vi "Solver.vi"(10 "Word List":string[](array[string]), 11 "Word Search Grid":string[][](array[string])) -> (3 "Solutions":T1)   [LabVIEW 2023]
uses:
  support/Solutions--map.ctl
  support/Letter Index--cluster.ctl
panel:
  # "Implement your Word Search challenge solution in this VI. Do not change the connector pane of this VI."
  # "Letters will always be ALL CAPS."
  # "Words will always be ALL CAPS."
  # "The Word Search Grid contains the 2D array of letters in which all words in the Word List appear. Words can appear forwards, backwards, up, down, and diagonally in any direction.\n\nThe Solutions map will contain one entry per item in the Word List. The map elements are:\n\nWord: The word from the Word List.\nLetter Indices: The row/column indices into the Word Search Grid for each letter (in order) in the word."
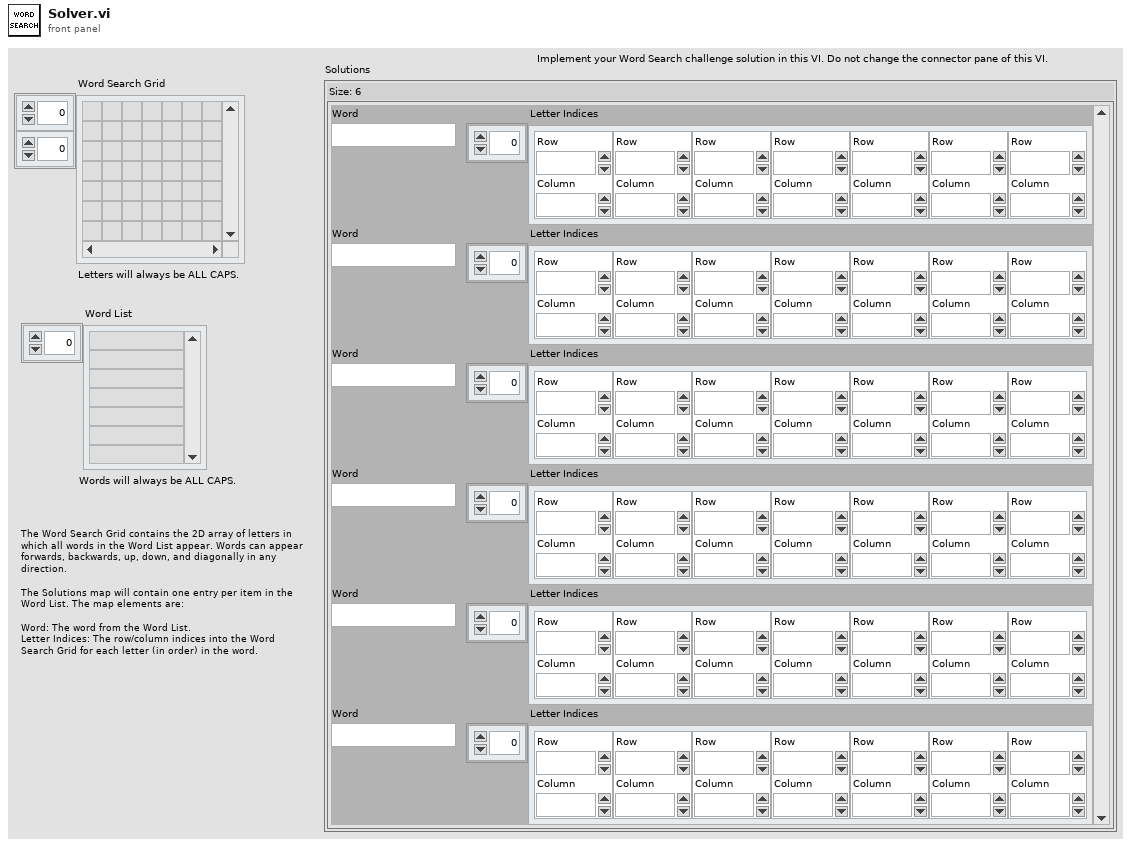
[diagram p1: front panel]
types:
  T1 = typedef "Solutions--map.ctl" = map{string, T2[]}
  T2 = typedef "Letter Index--cluster.ctl" = cluster{"Row":i32, "Column":i32}
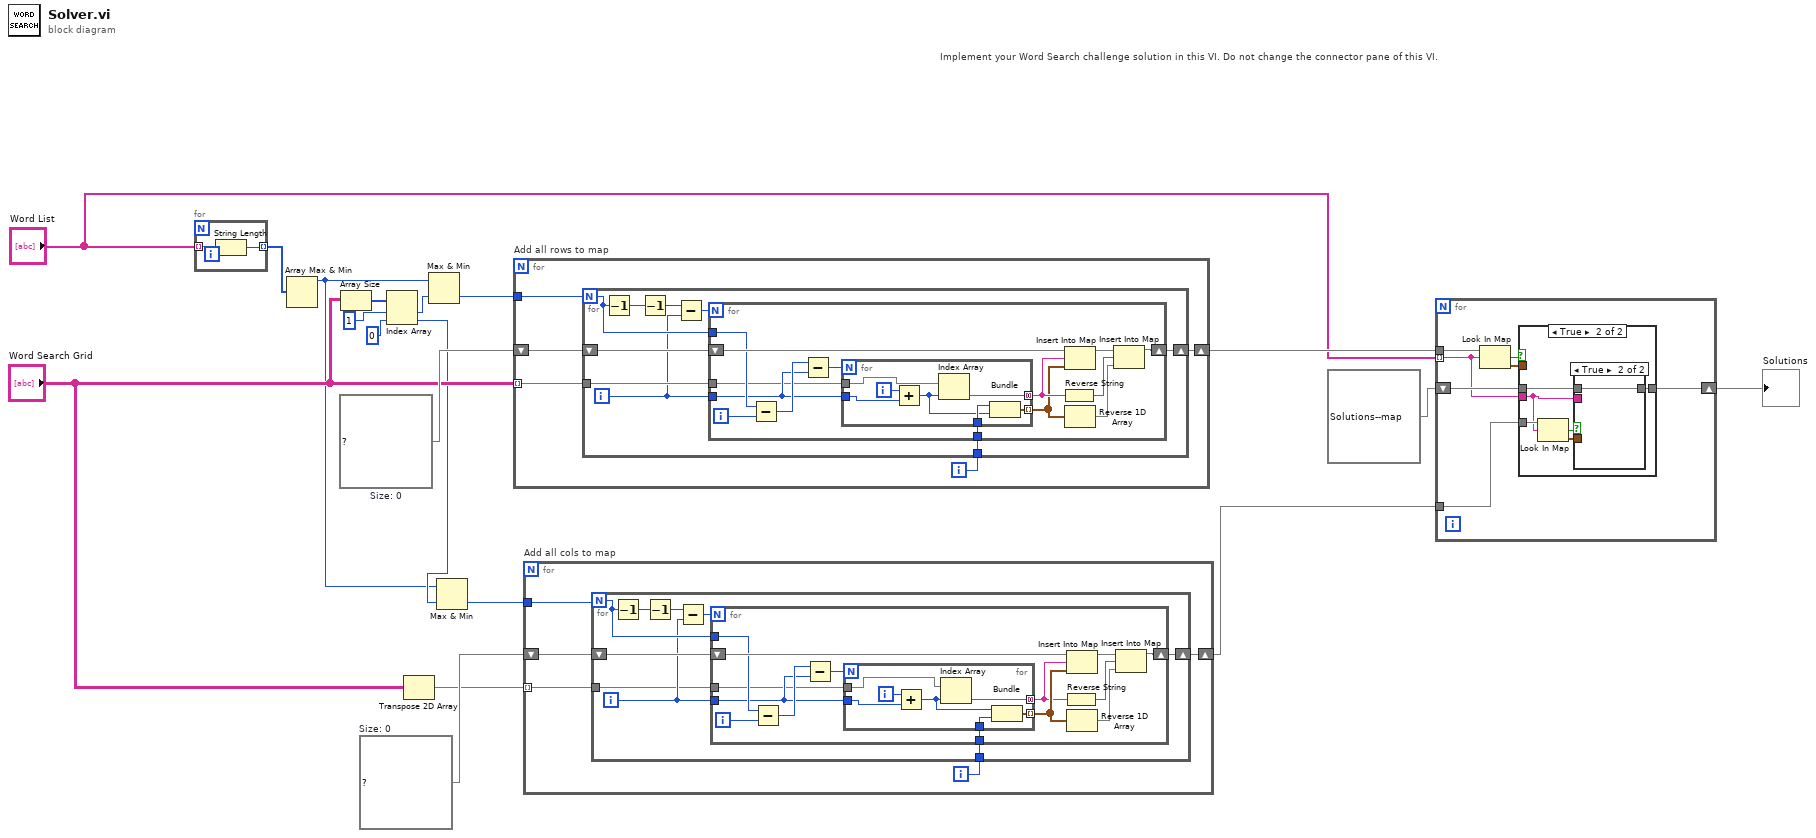
[diagram p0: block diagram]
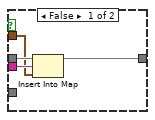
[diagram p2: hidden frame]
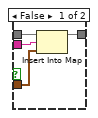
[diagram p3: hidden frame]
diagram:
  w13 = map{string, T2[]} {}  # Size: 0
  w17 = map{string, T2[]} {}  # Size: 0
  # "Implement your Word Search challenge solution in this VI. Do not change the connector pane of this VI."
  n1 = for {
    tunnel: "Word List" -> [w20] mode=indexing
    tunnel: [w19] -> w18 mode=indexing
    n2 = String Length(string=w20) -> (length=w19:i32)
  }
  n3 = Array Max & Min(array=w18) -> (max value=w3:i32)  [unwired: 3 out]
  n4 = Array Size(array="Word Search Grid") -> (size(s)=w11:i32[])
  n5 = Index Array(array=w11, index #1=1 ("index"), index #2=0 ("index")) -> (element #1=w9:i32, element #2=w4:i32)
  n6 = Transpose 2D Array(2D array="Word Search Grid") -> (transposed array=w2:string[][])
  n7 = Max & Min(x=w3, y=w9) -> (min(x,y)=w10:i32)  [unwired: 1 out]
  n8 = Max & Min(x=w3, y=w4) -> (min(x,y)=w5:i32)  [unwired: 1 out]
  n9 = for "Add all rows to map" {
    shift-right: [w24] -> w16
    shift-left: w17 -> [w25]
    tunnel: "Word Search Grid" -> [w23] mode=indexing
    tunnel: w10 -> [w21]
    i -> [w22]
    n10 = for {
      N: w21 -> [w30]
      tunnel: w23 -> [w34]
      shift-right: [w32] -> w24
      shift-left: w25 -> [w33]
      tunnel: w22 -> [w27]
      i -> [w28]
      n11 = Decrement(x=w30) -> (x-1=w31:i32)
      n12 = Decrement(x=w31) -> (x-1=w26:i32)
      n13 = Subtract(x=w26, y=w28) -> (x-y=w29:i32)
      n14 = for {
        N: w29 -> [_]
        tunnel: w34 -> [w40]
        shift-right: [w43] -> w32
        shift-left: w33 -> [w48]
        tunnel: w28 -> [w41]
        tunnel: w30 -> [w45]
        tunnel: w27 -> [w39]
        i -> [w46]
        n15 = Subtract(x=w45, y=w46) -> (x-y=w47:i32)
        n16 = Subtract(x=w47, y=w41) -> (x-y=w42:i32)
        n17 = for {
          N: w42 -> [_]
          tunnel: w41 -> [w54]
          tunnel: w40 -> [w53]
          tunnel: [w52] -> w38 mode=concatenating
          tunnel: w39 -> [w51]
          tunnel: [w49] -> w36 mode=indexing
          i -> [w55]
          n18 = Add(x=w55, y=w54) -> (x+y=w50:i32)
          n19 = Index Array(array=w53, index=w50) -> (element=w52:string)
          n20 = Bundle(w51, w50) -> (w49:cluster{i32, i32})  [unwired: 1 in]
        }
        n21 = Reverse String(1:w38) -> (0:w37:string)
        n22 = Insert Into Map(map in=w48, key=w38, value=w36) -> (map out=w44:map{string, T2[]})  [unwired: 2 out]
        n23 = Reverse 1D Array(array=w36) -> (reversed array=w35:cluster{i32, i32}[])
        n24 = Insert Into Map(map in=w44, key=w37, value=w35) -> (map out=w43:map{string, T2[]})  [unwired: 2 out]
      }
    }
  }
  n25 = for "Add all cols to map" {
    shift-right: [w59] -> w1
    shift-left: w13 -> [w60]
    tunnel: w5 -> [w57]
    tunnel: w2 -> [w56] mode=indexing
    i -> [w58]
    n26 = for {
      N: w57 -> [w66]
      shift-right: [w68] -> w59
      shift-left: w60 -> [w69]
      tunnel: w58 -> [w63]
      tunnel: w56 -> [w62]
      i -> [w64]
      n27 = Decrement(x=w66) -> (x-1=w67:i32)
      n28 = Decrement(x=w67) -> (x-1=w61:i32)
      n29 = Subtract(x=w61, y=w64) -> (x-y=w65:i32)
      n30 = for {
        N: w65 -> [_]
        shift-right: [w78] -> w68
        shift-left: w69 -> [w83]
        tunnel: w64 -> [w76]
        tunnel: w66 -> [w80]
        tunnel: w63 -> [w75]
        tunnel: w62 -> [w71]
        i -> [w81]
        n31 = Subtract(x=w80, y=w81) -> (x-y=w82:i32)
        n32 = Subtract(x=w82, y=w76) -> (x-y=w77:i32)
        n33 = for {
          N: w77 -> [_]
          tunnel: w76 -> [w89]
          tunnel: w75 -> [w84]
          tunnel: [w88] -> w73 mode=indexing
          tunnel: w71 -> [w87]
          tunnel: [w86] -> w70 mode=concatenating
          i -> [w90]
          n34 = Add(x=w90, y=w89) -> (x+y=w85:i32)
          n35 = Index Array(array=w87, index=w85) -> (element=w86:string)
          n36 = Bundle(w85, w84) -> (w88:cluster{i32, i32})  [unwired: 1 in]
        }
        n37 = Reverse String(1:w70) -> (0:w74:string)
        n38 = Insert Into Map(map in=w83, key=w70, value=w73) -> (map out=w79:map{string, T2[]})  [unwired: 2 out]
        n39 = Reverse 1D Array(array=w73) -> (reversed array=w72:cluster{i32, i32}[])
        n40 = Insert Into Map(map in=w79, key=w74, value=w72) -> (map out=w78:map{string, T2[]})  [unwired: 2 out]
      }
    }
  }
  n41 = for {
    tunnel: "Word List" -> [w92] mode=indexing
    tunnel: w16 -> [w97]
    shift-right: [w91] -> w14
    shift-left: T1 {} ("Solutions") -> [w96]
    tunnel: w1 -> [w93]
    n42 = Look In Map(map=w97, key=w92) -> (key not found?=w94:bool, value=w95:T2[])  [unwired: 1 in]
    n43 = case shown="True" w94 {
      tunnel: w96 -> [w101 w104]
      tunnel: w92 -> [w100 w102]
      tunnel: w95 -> [w99 _]
      tunnel: [w98 w103] -> w91
      tunnel: w93 -> [_ w107]
      frame False {
        n44 = Insert Into Map(map in=w101, key=w100, value=w99) -> (map out=w98:T1)  [unwired: 2 out]
      }
      frame True {
        n45 = Look In Map(map=w107, key=w102) -> (key not found?=w106:bool, value=w105:T2[])  [unwired: 1 in]
        n46 = case shown="True" w106 {
          tunnel: w105 -> [w108 _]
          tunnel: w104 -> [w111 w112]
          tunnel: [w110 w112] -> w103
          tunnel: w102 -> [w109 _]
          frame False {
            n47 = Insert Into Map(map in=w111, key=w109, value=w108) -> (map out=w110:T1)  [unwired: 2 out]
          }
          frame True {
          }
        }
      }
    }
  }
  "Solutions" <- w14
